vi "init_camCorrection.vi"(8 "error in":errorcluster, 10 "orig image":T3, 11 "cam info in":T1={"camera type"=enum."Qcam", "cam handle"=0, "data handle"=0, "cam size"=[]}) -> (0 "error out":errorcluster, 2 "orig image out":T3)   [LabVIEW 2015]
uses:
  <vilib>/vision/Image Controls.llb/IMAQ Image.ctl
  controls/cam_info.ctl
  controls/cam_type-v02.ctl
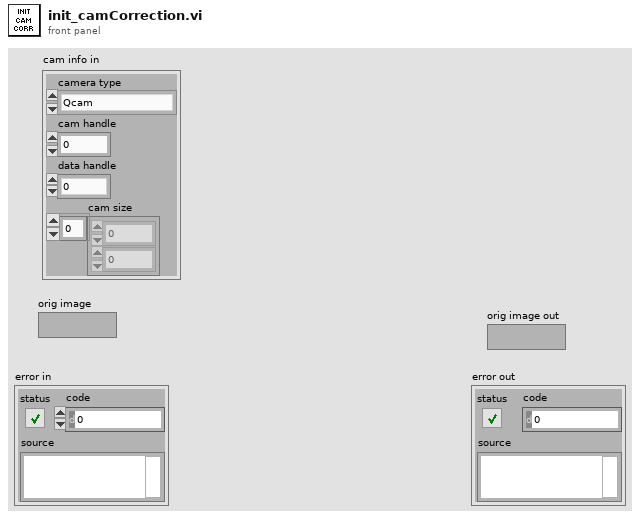
[diagram p1: front panel]
types:
  T1 = typedef "cam_info.ctl" = cluster{"camera type":T2, "cam handle":u32, "data handle":u32, "cam size":i32[]}
  T2 = typedef "cam_type-v02.ctl" = enum16{"HamamatsuORCA05G", "Qcam", "optiMOS"}
  T3 = typedef "IMAQ Image.ctl" = refnum<image>
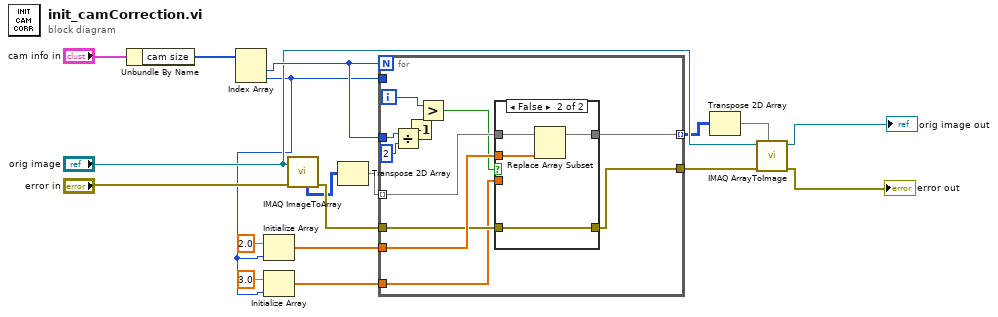
[diagram p0: block diagram]
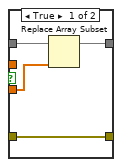
[diagram p2: hidden frame]
diagram:
  n1 = Unbundle By Name("cam info in") -> ("cam size"=w17:i32[])
  n2 = Index Array(array=w17) -> (element #1=w13:i32, element #2=w4:i32)  [unwired: 2 in]
  n3 = Initialize Array(2.0 ("element"), w4) -> (w6:dbl[])
  n4 = Initialize Array(3.0 ("element"), w4) -> (w3:dbl[])
  n5 = call "IMAQ ImageToArray"("error in (no error)"="error in", "Image"="orig image") -> ("Image Pixels (U16)"=w9:u16[][], "error out"=w11:errorcluster)  [unwired: 2 in, 3 out]
  n6 = Transpose 2D Array(2D array=w9) -> (transposed array=w8:u16[][])
  n7 = for {
    N: w13 -> [_]
    tunnel: w4 -> [_]
    tunnel: w13 -> [w24]
    tunnel: w8 -> [w30] mode=indexing
    tunnel: [w29] -> w2 mode=indexing
    tunnel: w11 -> [w27]
    tunnel: [w26] -> w10
    tunnel: w6 -> [w28]
    tunnel: w3 -> [w25]
    i -> [w21]
    n8 = Divide(x=w24, y=2) -> (x/y=w22:dbl)
    n9 = Decrement(x=w22) -> (x-1=w19:dbl)
    n10 = Greater?(x=w21, y=w19) -> (0:w20:bool)
    n11 = case shown="False" w20 {
      tunnel: w30 -> [w34 w38]
      tunnel: [w33 w37] -> w29
      tunnel: w28 -> [_ w35]
      tunnel: w27 -> [w32 w36]
      tunnel: [w32 w36] -> w26
      tunnel: w25 -> [w31 _]
      frame True {
        n12 = Replace Array Subset(array=w34, new element=w31) -> (w33:u16[])  [unwired: 1 in]
      }
      frame False {
        n13 = Replace Array Subset(array=w38, new element=w35) -> (w37:u16[])  [unwired: 1 in]
      }
    }
  }
  n14 = Transpose 2D Array(2D array=w2) -> (transposed array=w1:u16[][])
  n15 = call "IMAQ ArrayToImage"("Image Pixels (U16)"=w1, "error in (no error)"=w10, "Image"="orig image") -> ("error out"=→"error out":errorcluster, "Image Out"=→"orig image out":T3)  [unwired: 7 in]
